vi "AlazarSetTriggerDelay.vi"(3 "error in (no error)":errorcluster, 4 "Delay":u32, 5 "Handle":u64) -> (0 "error out":errorcluster, 1 "Return Code":u32, 2 "Handle":u64)   [LabVIEW 2018]
doc: "Set the time, in sample clocks, to wait after receiving a trigger event before capturing a record for the trigger."
uses:
  ATSApi.dll
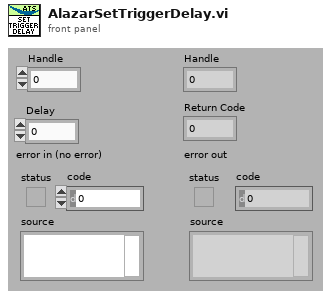
[diagram p1: front panel]
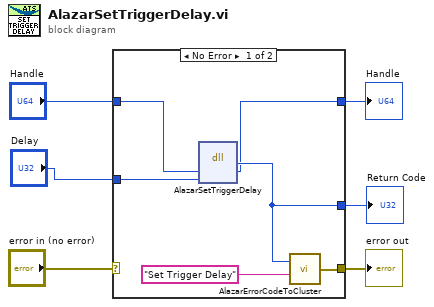
[diagram p0: block diagram]
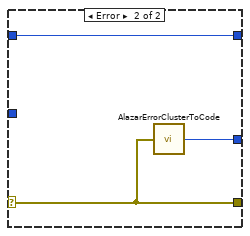
[diagram p2: hidden frame]
diagram:
  n1 = case shown="No Error" "error in (no error)" {
    selector: "error in (no error)" -> [_ w15]
    tunnel: [w9 w15] -> w5
    tunnel: [w11 w14] -> w4
    tunnel: "Handle" -> [w12 w13]
    tunnel: [w8 w13] -> w2
    tunnel: "Delay" -> [w7 _]
    frame No Error {
      n2 = dll-call lib="ATSApi.dll" fn="AlazarSetTriggerDelay"("handle"=w12, "value"=w7) -> ("return type"=w11:u32, "handle"=w8:u64)  [unwired: 4 in, 2 out]
      n3 = call "AlazarErrorCodeToCluster.vi"("Message"="Set Trigger Delay", "Error Code"=w11) -> ("error out"=w9:errorcluster)
    }
    frame Error {
      n4 = call "AlazarErrorClusterToCode.vi"("error in (no error)"=w15) -> ("Error Code"=w14:u32)
    }
  }
  "Handle" <- w2
  "error out" <- w5
  "Return Code" <- w4
